vi "readCO2Levels.vi"(8 "error in (no error)":errorcluster, 11 "VISA resource name":refnum<visa-resource-name>) -> (0 "error IO":errorcluster, 2 "Fast Level":i32, 3 "Filtered Level":i32)   [LabVIEW 2013]
uses:
  <vilib>/regexp/Match Regular Expression.xnode
panel:
  out "read buffer":string
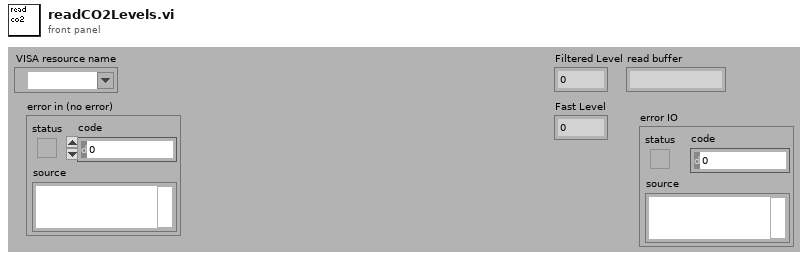
[diagram p1: front panel]
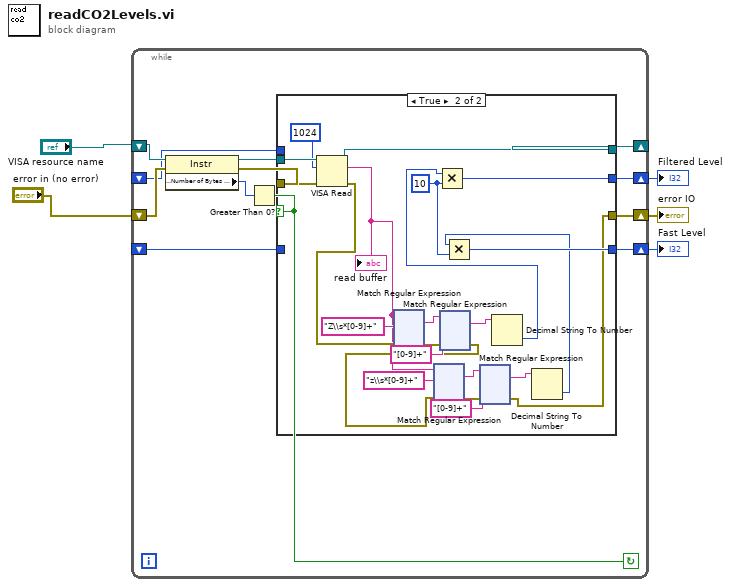
[diagram p0: block diagram]
diagram:
  n1 = while {
    shift-right: [w12] -> _
    shift-left: "VISA resource name" -> [w17]
    shift-right: [w11] -> w3
    shift-left: _ -> [w7]
    shift-right: [w10] -> w2
    shift-left: _ -> [w6]
    shift-right: [w9] -> w1
    shift-left: "error in (no error)" -> [w8]
    stop <- w13 continue-if-true
    n2 = property class="Instr"(reference=w17, error in=w8) -> (reference out=w16:refnum<visa-resource-name>, error out=w15:errorcluster, "Serial Settings:Number of Bytes at Serial Port"=w14:u32)
    n3 = Greater Than 0?(x=w14) -> (x > 0?=w13:bool)
    n4 = case shown="True" w13 {
      tunnel: w16 -> [w20 w44]
      tunnel: w15 -> [w18 w43]
      tunnel: [w18 w26] -> w9
      tunnel: [w20 w42] -> w12
      tunnel: [w21 w41] -> w11
      tunnel: [w19 w39] -> w10
      tunnel: w7 -> [w21 _]
      tunnel: w6 -> [w19 _]
      frame False {
      }
      frame True {
        w40 = 10 ("y")
        n5 = VISA Read(VISA resource name=w44, byte count=u32 1024, error in (no error)=w43) -> (VISA resource name out=w42:refnum<visa-resource-name>, read buffer=w23:string, error out=w35:errorcluster)  [unwired: 1 out]
        "read buffer" <- w23
        n6 = xnode "Match Regular Expression"("input string"=w23, "regular expression"="Z\\s*[0-9]+", "error in"=w35) -> ("whole match"=w37:string, "error out"=w36:errorcluster)  [unwired: 3 in, 3 out]
        n7 = xnode "Match Regular Expression"("input string"=w37, "regular expression"="[0-9]+", "error in"=w36) -> ("whole match"=w33:string, "error out"=w25:errorcluster)  [unwired: 3 in, 3 out]
        n8 = xnode "Match Regular Expression"("input string"=w23, "regular expression"="z\\s*[0-9]+", "error in"=w25) -> ("whole match"=w30:string, "error out"=w29:errorcluster)  [unwired: 3 in, 3 out]
        n9 = xnode "Match Regular Expression"("input string"=w30, "regular expression"="[0-9]+", "error in"=w29) -> ("whole match"=w27:string, "error out"=w26:errorcluster)  [unwired: 3 in, 3 out]
        n10 = Decimal String To Number(string=w33) -> (number=w32:i32)  [unwired: 2 in, 1 out]
        n11 = Multiply(x=w32, y=w40) -> (x*y=w41:i32)
        n12 = Decimal String To Number(string=w27) -> (number=w24:i32)  [unwired: 2 in, 1 out]
        n13 = Multiply(x=w24, y=w40) -> (x*y=w39:i32)
      }
    }
  }
  "Filtered Level" <- w3
  "Fast Level" <- w2
  "error IO" <- w1
